vi "Build Project.vi"(8 "error in (no error)":errorcluster, 11 "Project Path":path) -> (0 "error out":errorcluster, 1 "Success?":bool, 3 "Report Array":refnum<class "Report Data.lvclass">[](array[class]))   [LabVIEW 2020, in "ProjectBuilder.lvlib"]
uses:
  ProjectBuilder.lvlib
  Class/Data/Report Data/Report Data.lvclass
  Sub/Private/Ctl/Ctl_Build Steps.ctl
  Class/Report Action/Report Action/Report Action.lvclass/Report Action.ctl
  Class/Report Action/Report Action/Report Action.lvclass
  C:/Current projects/WS/LV32.2020..ProjectBuilder/Class/Action/Project Action/Project Action.lvclass
  <vilib>/Utility/error.llb/Error Cluster From Error Code.vi
  <vilib>/ErrorRing/Error Ring.xnode
  <vilib>/Utility/Data Type/NI_Data Type.lvlib
  PPL/HDH.ClassLoader.lvlibp
  Class/Action/Project Action/Project Action.lvclass
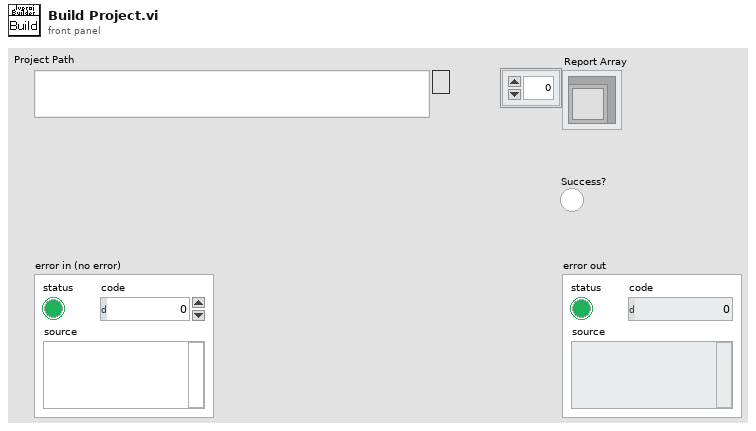
[diagram p1: front panel]
types:
  T1 = typedef "ProjectBuilder.lvlib/Ctl_Build Steps.ctl" = enum16{"Source Test", "Build", "Post-Build Test", "Deploy", "Report"}
  T2 = typedef "ProjectBuilder.lvlib/Ctl_Run Cluster.ctl" = cluster{"Source Tests":refnum<class "Project Action.lvclass">[], "Build Array":refnum<class "Project Action.lvclass">[], "Post-Build Tests":refnum<class "Project Action.lvclass">[], "Deploy Array":refnum<class "Project Action.lvclass">[], "Report Handler Array":refnum<class "Report Action.lvclass">[]}
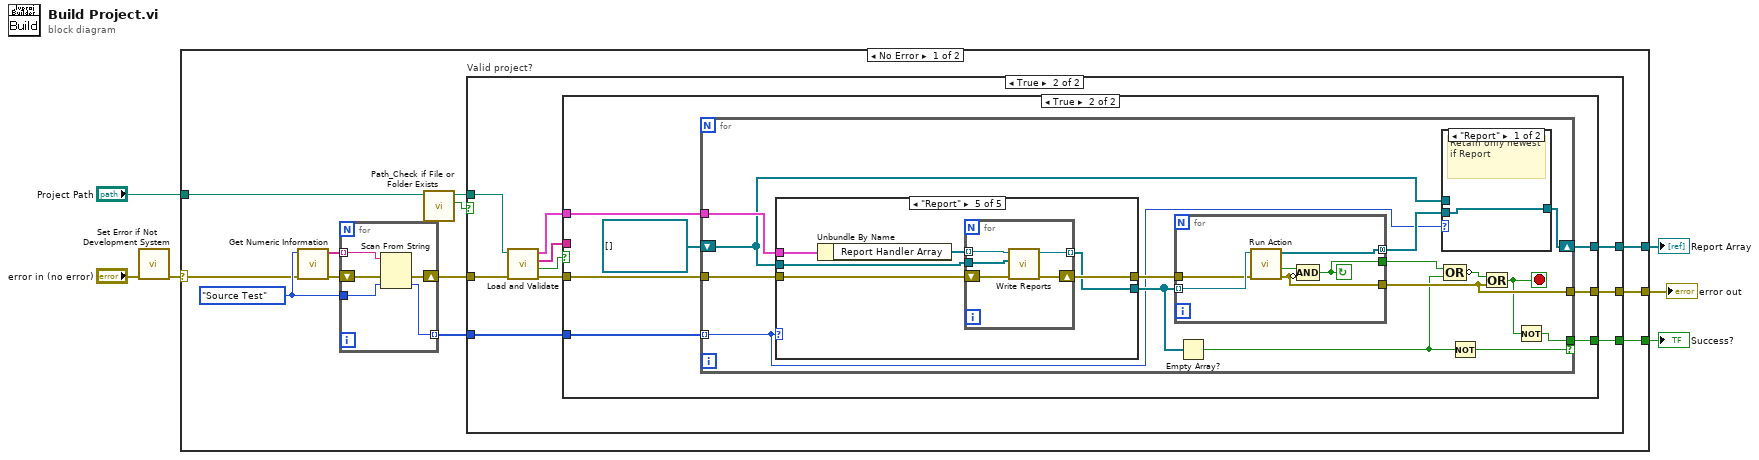
[diagram p0: block diagram]
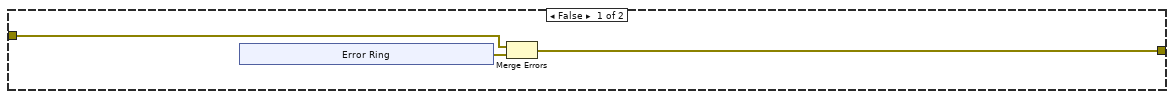
[diagram p2: hidden frame]
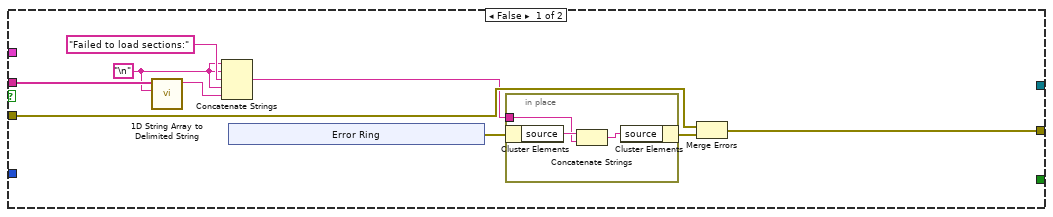
[diagram p3: hidden frame]
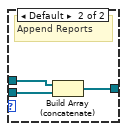
[diagram p4: hidden frame]
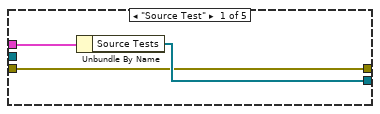
[diagram p5: hidden frame]
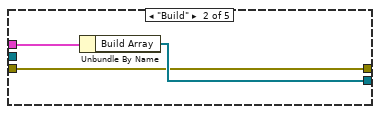
[diagram p6: hidden frame]
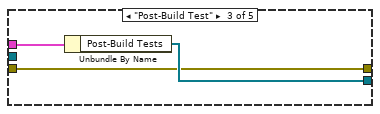
[diagram p7: hidden frame]
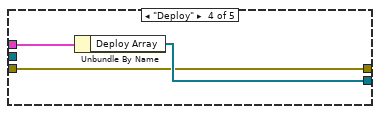
[diagram p8: hidden frame]
diagram:
  n1 = call "Set Error if Not Development System.vi"("error in (no error)"="error in (no error)") -> ("error out"=w3:errorcluster)  [unwired: 10 in]
  n2 = case shown="No Error" w3 {
    selector: w3 -> [w13 w112]
    tunnel: "Project Path" -> [w14 _]
    tunnel: [w9 w112] -> w5
    tunnel: [w8 _] -> w2
    tunnel: [w7 _] -> w1
    frame No Error {
      w18 = Ctl_Build_Steps."Source Test" ("Build Step")
      n3 = call <vilib>:"Get Numeric Information.vi"("error in (no error)"=w13, "variant"=w18) -> ("error out"=w16:errorcluster, "enum names"=w17:string[])  [unwired: 6 in, 2 out]
      n4 = for {
        tunnel: w18 -> [w111]
        tunnel: w17 -> [w110] mode=indexing
        tunnel: [w109] -> w15 mode=indexing
        shift-right: [w107] -> w11
        shift-left: w16 -> [w108]
        n5 = Scan From String(input string=w110, error in=w108, default 1=w111) -> (error out=w107:errorcluster, output 1=w109:T1)  [unwired: 2 in, 2 out]
      }
      n6 = call "Path_Check if File or Folder Exists.vi"("File or Folder Path in"=w14) -> ("File or Folder Found?"=w12:bool, "File or Folder Path dub"=w10:path)  [unwired: 9 in]
      n7 = case "Valid project?" shown="True" w12 {
        tunnel: w15 -> [_ w35]
        tunnel: [w19 w34] -> w9
        tunnel: w11 -> [w21 w31]
        tunnel: w10 -> [_ w33]
        tunnel: [_ w27] -> w8
        tunnel: [_ w26] -> w7
        frame False {
          n8 = xnode "Error Ring"() -> ("error out"=w20:errorcluster)
          n9 = Merge Errors(w21, w20) -> (w19:errorcluster)
        }
        frame True {
          n10 = call "Load and Validate.vi"("error in (no error)"=w31, "Project Path"=w33) -> ("error out"=w32:errorcluster, "Valid?"=w29:bool, "Invalid Sections"=w28:string[], "Run cluster"=w30:T2)  [unwired: 6 in]
          n11 = case shown="True" w29 {
            tunnel: w35 -> [_ w58]
            tunnel: [w43 w55] -> w34
            tunnel: w32 -> [w44 w57]
            tunnel: w30 -> [_ w56]
            tunnel: w28 -> [w40 _]
            tunnel: [_ w53] -> w27
            tunnel: [_ w52] -> w26
            frame False {
              w36 = "\n"
              n12 = call <vilib>:"1D String Array to Delimited String.vi"("delimiter"=w36, "string array"=w40) -> ("delimited string"=w38:string)  [unwired: 9 in]
              n13 = Concatenate Strings(w36, w36, "Failed to load sections:", w36, w38) -> (w37:string)
              n14 = xnode "Error Ring"() -> ("error out"=w42:errorcluster)
              n15 = in-place {
                in-place-border: w37 -> [w46]
                n16 = in-place-cluster #1(w42) -> ("source"=w47:string)
                n17 = Concatenate Strings(w47, w46) -> (w45:string)
                n18 = in-place-cluster #1("source"=w45) -> (w41:errorcluster)
              }
              n19 = Merge Errors(w44, w41) -> (w43:errorcluster)
            }
            frame True {
              n20 = for {
                tunnel: w58 -> [w63] mode=indexing
                tunnel: w57 -> [w64]
                tunnel: [w72] -> w55
                tunnel: w56 -> [w73]
                shift-right: [w67] -> w53
                shift-left: refnum<class "Report Data.lvclass">[] [] ("Report Array") -> [w66]
                tunnel: [w59] -> w52 if=w60
                stop <- w62 stop-if-true
                n21 = case shown="\"Report\"" w63 {
                  tunnel: w73 -> [w86 w89 w92 w95 w101]
                  tunnel: [w85 w88 w91 w94 w96] -> w71
                  tunnel: w66 -> [_ _ _ _ w99]
                  tunnel: w64 -> [w84 w87 w90 w93 w98]
                  tunnel: [w84 w87 w90 w93 w97] -> w65
                  frame "Source Test" {
                    n22 = Unbundle By Name(w86) -> ("Source Tests"=w85:refnum<class "Project Action.lvclass">[])
                  }
                  frame "Build" {
                    n23 = Unbundle By Name(w89) -> ("Build Array"=w88:refnum<class "Project Action.lvclass">[])
                  }
                  frame "Post-Build Test" {
                    n24 = Unbundle By Name(w92) -> ("Post-Build Tests"=w91:refnum<class "Project Action.lvclass">[])
                  }
                  frame "Deploy" {
                    n25 = Unbundle By Name(w95) -> ("Deploy Array"=w94:refnum<class "Project Action.lvclass">[])
                  }
                  frame "Report" {
                    n26 = Unbundle By Name(w101) -> ("Report Handler Array"=w100:refnum<class "Report Action.lvclass">[])
                    n27 = for {
                      tunnel: w100 -> [w106] mode=indexing
                      tunnel: w99 -> [w105]
                      shift-right: [w103] -> w97
                      shift-left: w98 -> [w104]
                      tunnel: [w102] -> w96 mode=indexing
                      n28 = call "Write Reports.vi"("error in (no error)"=w104, "Reports"=w105, "Report Action in"=w106) -> ("error out"=w103:errorcluster, "Report Action out"=w102:refnum<class "Report Action.lvclass">)  [unwired: 7 in]
                    }
                  }
                }
                n29 = for {
                  tunnel: w71 -> [w83] mode=indexing
                  tunnel: w65 -> [w82]
                  tunnel: [w80] -> w68 mode=concatenating
                  tunnel: [w79] -> w72
                  tunnel: [w78] -> w70
                  stop <- w78 continue-if-true
                  n30 = call "Run Action.vi"("error in (no error)"=w82, "Project Action"=w83) -> ("error out"=w79:errorcluster, "Success?"=w81:bool, "Report Array"=w80:refnum<class "Report Data.lvclass">[])  [unwired: 7 in]
                  n31 = Compound Arithmetic op=AND(w81, invert w79) -> (w78:bool)
                }
                n32 = Empty Array?(array=w71) -> (empty?=w61:bool)
                n33 = case shown="\"Report\"" w63 {
                  tunnel: w68 -> [w74 w77]
                  tunnel: [w74 w76] -> w67
                  tunnel: w66 -> [_ w75]
                  frame "Report" {
                    # "Retain only newest if Report"
                  }
                  frame Default {
                    # "Append Reports"
                    n34 = Build Array (concatenate)(w75, w77) -> (w76:refnum<class "Report Data.lvclass">[])
                  }
                }
                n35 = Compound Arithmetic op=OR(w70, w61) -> (invert w69:bool)
                n36 = Not(x=w61) -> (.not. x?=w60:bool)
                n37 = Or(x=w69, y=w72) -> (x .or. y?=w62:bool)
                n38 = Not(x=w62) -> (.not. x?=w59:bool)
              }
            }
          }
        }
      }
    }
    frame Error {
    }
  }
  "error out" <- w5
  "Report Array" <- w2
  "Success?" <- w1
